vi "GetDEMUXStatus.vi"(11 "Input String":string) -> (3 "DEMUX status":bool[](array[boolean]))   [LabVIEW 2012]
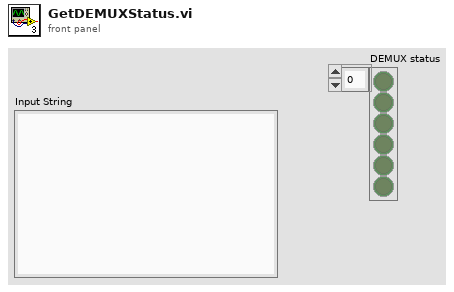
[diagram p1: front panel]
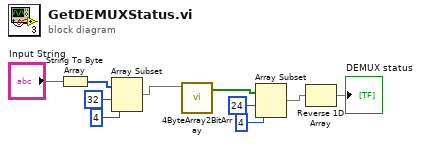
[diagram p0: block diagram]
diagram:
  n1 = String To Byte Array(string="Input String") -> (unsigned byte array=w9:u8[])
  n2 = Array Subset(array=w9, index=32, length=4) -> (w5:u8[])
  n3 = call "4ByteArray2BitArray.vi"("array"=w5) -> ("Array"=w10:bool[])  [unwired: 10 in]
  n4 = Array Subset(array=w10, index=24, length=4) -> (w8:bool[])
  n5 = Reverse 1D Array(array=w8) -> (reversed array=→"DEMUX status":bool[])
